vi "只找到一个缺口时-利用圆心算出相对的另一个缺口.vi"(8 "每个缺口像素点数量":i32[](array[numeric])=[11, 5, 12], 9 "Fitted Circle":T3, 10 "存储缺口位置in":cluster{"X":sgl, "Y":sgl}[](array[cluster]), 11 "img in":T2) -> (1 "存储缺口位置 out":cluster{"X":sgl, "Y":sgl}[](array[cluster]), 3 "img out":T2)   [LabVIEW 2014]
uses:
  <vilib>/vision/Image Controls.llb/IMAQ Image.ctl
panel:
  out "最小值":dbl
  out "数组 2":dbl[](array[numeric])
  out "数组":T1(array[cluster])
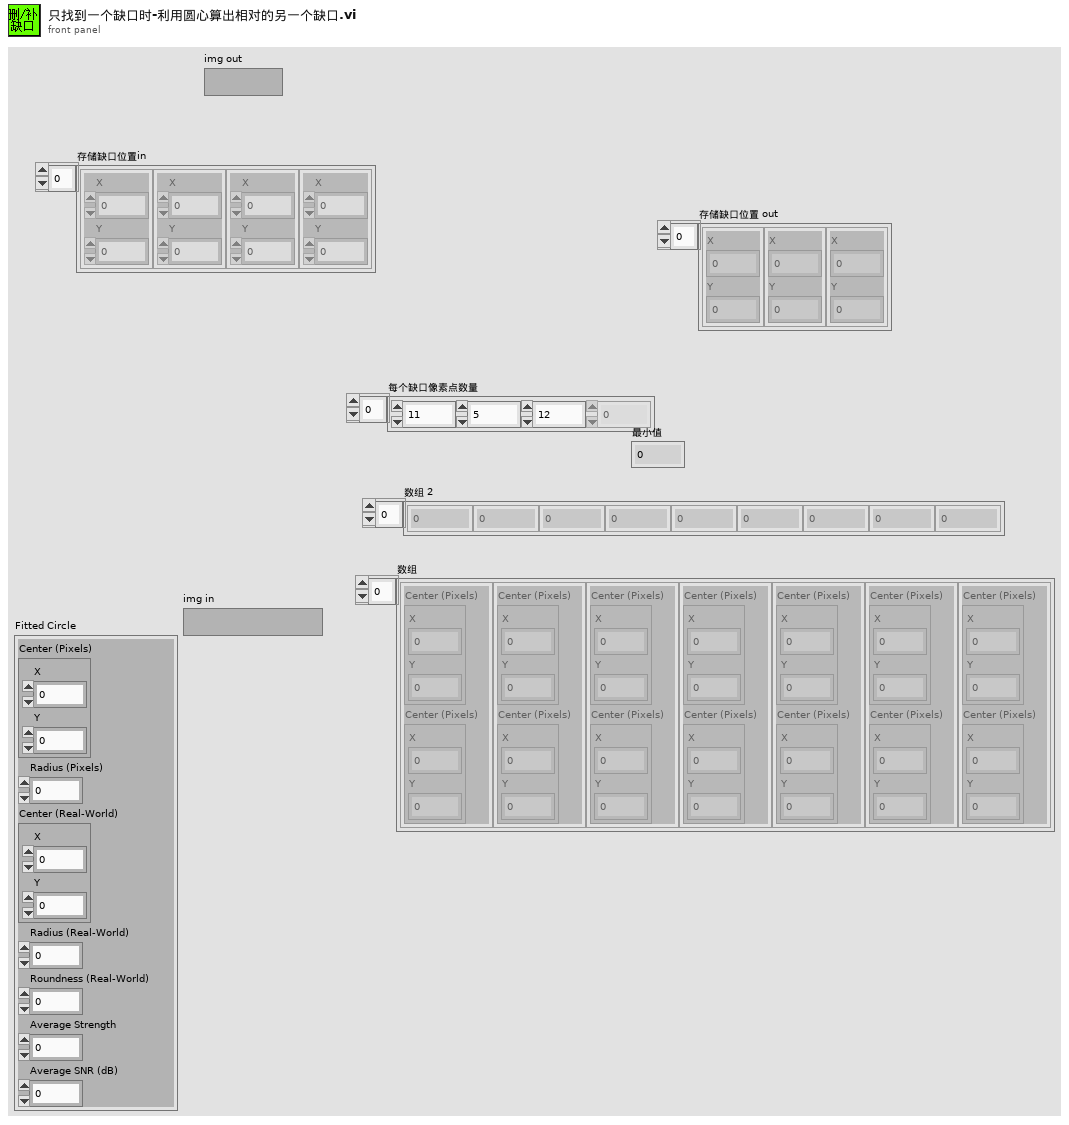
[diagram p1: front panel]
types:
  T1 = cluster{"Center (Pixels)":cluster{"X":sgl, "Y":sgl}, "Center (Pixels)":cluster{"X":sgl, "Y":sgl}}[]
  T2 = typedef "IMAQ Image.ctl" = refnum<image>
  T3 = cluster{"Center (Pixels)":cluster{"X":sgl, "Y":sgl}, "Radius (Pixels)":dbl, "Center (Real-World)":cluster{"X":sgl, "Y":sgl}, "Radius (Real-World)":dbl, "Roundness (Real-World)":dbl, "Average Strength":dbl, "Average SNR (dB)":dbl}
  T4 = cluster{"Center (Pixels)":cluster{"X":sgl, "Y":sgl}, "Center (Pixels)":cluster{"X":sgl, "Y":sgl}}
  T5 = cluster{"存储缺口位置in[0]":cluster{"X":dbl, "Y":dbl}, "存储缺口位置in[1]":cluster{"X":dbl, "Y":dbl}}
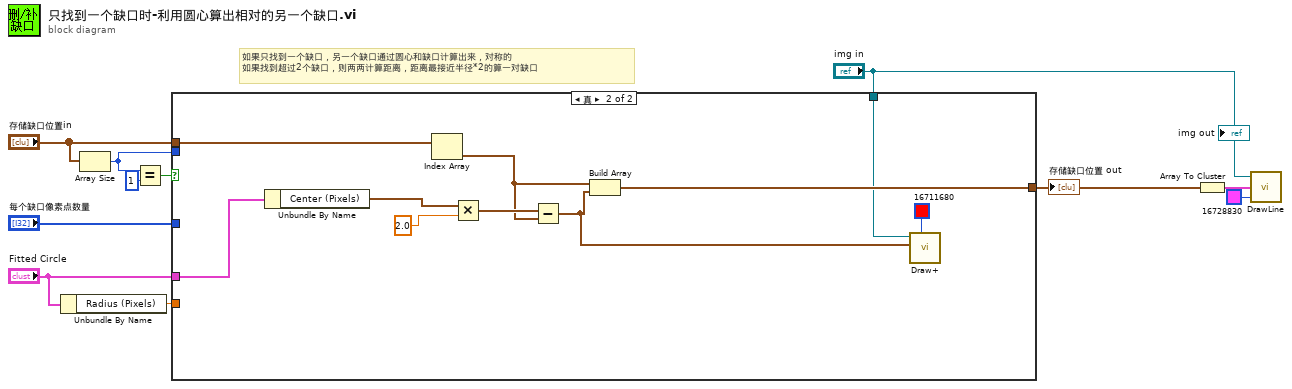
[diagram p0: block diagram]
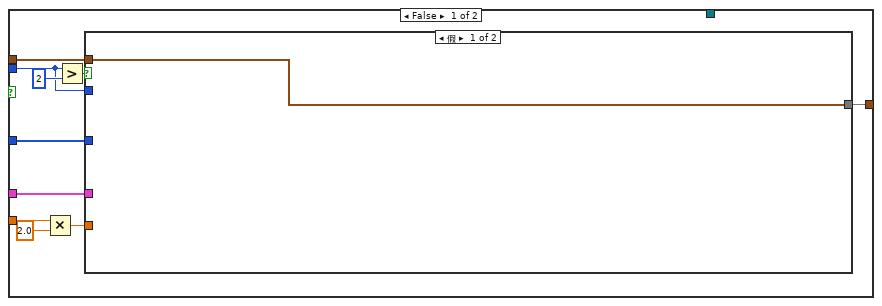
[diagram p2: hidden frame]
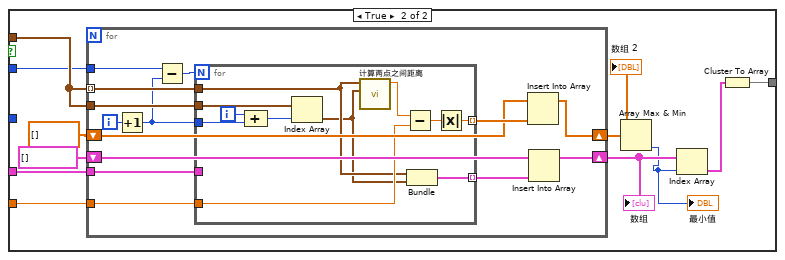
[diagram p3: hidden frame]
diagram:
  # "如果只找到一个缺口，另一个缺口通过圆心和缺口计算出来，对称的\n如果找到超过2个缺口，则两两计算距离，距离最接近半径*2的算一对缺口"
  n1 = Unbundle By Name("Fitted Circle") -> ("Radius (Pixels)"=w2:dbl)
  n2 = Array Size(array="存储缺口位置in") -> (size(s)=w4:i32)
  n3 = Equal?(x=w4, y=1) -> (x = y?=w9:bool)
  n4 = case shown="真" w9 {
    tunnel: [w17 w64] -> w6
    tunnel: "存储缺口位置in" -> [w18 w63]
    tunnel: "每个缺口像素点数量" -> [w20 _]
    tunnel: w4 -> [w12 _]
    tunnel: "Fitted Circle" -> [w16 w62]
    tunnel: w2 -> [w15 _]
    tunnel: "img in" -> [_ w61]
    frame False {
      n5 = Multiply(x=w15, y=2.0) -> (x*y=w13:dbl)
      n6 = Greater?(x=w12, y=2) -> (0:w19:bool)
      n7 = case shown="假" w19 {
        tunnel: w20 -> [_ _]
        tunnel: w18 -> [w22 w33]
        tunnel: [w22 w26] -> w17
        tunnel: w16 -> [_ w32]
        tunnel: w13 -> [_ w31]
        tunnel: w12 -> [_ w25]
        frame False {
        }
        frame True {
          n8 = for {
            tunnel: w33 -> [w47]
            tunnel: w33 -> [w46] mode=indexing
            tunnel: w32 -> [w45]
            tunnel: w31 -> [w44]
            shift-right: [w41] -> w29
            shift-left: dbl[] [] -> [w42]
            shift-right: [w40] -> w28
            shift-left: T1 [] -> [w39]
            tunnel: w25 -> [w36]
            i -> [w37]
            n9 = Increment(x=w37) -> (x+1=w35:i32)
            n10 = Subtract(x=w36, y=w35) -> (x-y=w34:i32)
            n11 = for {
              N: w34 -> [_]
              tunnel: w47 -> [w56]
              tunnel: w46 -> [w50]
              tunnel: w35 -> [w57]
              tunnel: w45 -> [_]
              tunnel: w44 -> [w53]
              tunnel: [w51] -> w43 mode=indexing
              tunnel: [w48] -> w38 mode=indexing
              i -> [w58]
              n12 = Compound Arithmetic op=ADD(w58, w57) -> (w55:i32)
              n13 = Index Array(array=w56, index=w55) -> (element=w49:cluster{"X":sgl, "Y":sgl})
              n14 = call "计算两点之间距离.vi"("Location (Pixel)"=w49, "Center (Pixels)"=w50) -> ("两点之间距离"=w54:sgl)  [unwired: 9 in]
              n15 = Subtract(x=w54, y=w53) -> (x-y=w52:dbl)
              n16 = Bundle("Center (Pixels)"=w50, "Center (Pixels)"=w49) -> (w48:T4)  [unwired: 1 in]
              n17 = Absolute Value(x=w52) -> (abs(x)=w51:dbl)
            }
            n18 = Insert Into Array(array=w42, new element=w43) -> (w41:dbl[])  [unwired: 1 in]
            n19 = Insert Into Array(array=w39, new element=w38) -> (w40:T1)  [unwired: 1 in]
          }
          "数组" <- w28
          "数组 2" <- w29
          n20 = Array Max & Min(array=w29) -> (min index (indices)=w24:i32)  [unwired: 3 out]
          "最小值" <- w24
          n21 = Index Array(array=w28, index=w24) -> (element=w27:T4)
          n22 = Cluster To Array(cluster=w27) -> (array=w26:cluster{"X":sgl, "Y":sgl}[])
        }
      }
    }
    frame True {
      n23 = Unbundle By Name(w62) -> ("Center (Pixels)"=w68:cluster{"X":sgl, "Y":sgl})
      n24 = Index Array(array=w63) -> (element=w65:cluster{"X":sgl, "Y":sgl})  [unwired: 1 in]
      n25 = Multiply(x=w68, y=2.0) -> (x*y=w66:cluster{"X":dbl, "Y":dbl})
      n26 = Subtract(x=w66, y=w65) -> (x-y=w60:cluster{"X":dbl, "Y":dbl})
      n27 = Build Array(w65, w60) -> (w64:cluster{"X":dbl, "Y":dbl}[])
      n28 = call "Draw+.vi"("Color"=u32 16711680, "input cluster"=w60, "Image In"=w61) -> ()  [unwired: 3 in, 1 out]
    }
  }
  "存储缺口位置 out" <- w6
  n29 = Array To Cluster(array=w6) -> (cluster=w8:T5)
  n30 = call "DrawLine.vi"("Color"=u32 16728830, "Edge Points"=w8, "img in"="img in") -> ()  [unwired: 1 out]
  "img out" <- "img in"
